vi "集成干预测试数据存储.vi"(8 "error in (no error)":errorcluster, 11 "存储变量":T1) -> (0 "error out":errorcluster)   [LabVIEW 2016, in "PLC.lvlib"]
uses:
  PLC.lvlib
  <vilib>/Utility/sysdir.llb/System Directory Type.ctl
  <vilib>/addons/database/Connection.llb/DB Tools Open Connec (String).vi
  <vilib>/addons/database/NI_Database_API.lvlib
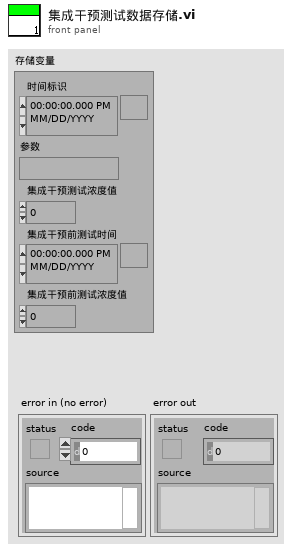
[diagram p1: front panel]
types:
  T1 = cluster{"时间标识":timestamp, "参数":string, "集成干预测试浓度值":dbl, "集成干预前测试时间":timestamp, "集成干预前测试浓度值":dbl}
  T2 = typedef "System Directory Type.ctl" = i32
  T3 = typedef "NI_Database_API.lvlib/Conn ObjectReference.ctl" = refnum<k1>
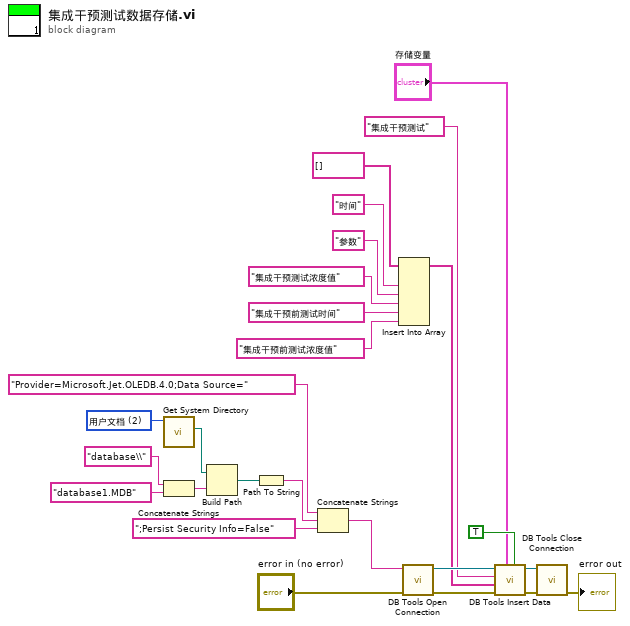
[diagram p0: block diagram]
diagram:
  w23 = T2 2 items=["用户目录"=0, "用户桌面"=1, "用户文档"=2, "用户应用程序数据"=3, "用户设置"=4, "用户临时目录"=5, "公共文档"=6, "公共应用程序数据"=7, "公共设置"=8, "公共缓存"=13, "系统核心库"=9, "系统安装库"=10, "应用程序文件"=11, "启动盘根目录"=12] ("system directory type")
  n1 = call <vilib>:"Get System Directory.vi"("system directory type"=w23) -> ("system directory"=w21:path)  [unwired: 10 in]
  n2 = Concatenate Strings("database\\" ("condition"), "database1.MDB" ("condition")) -> (w15:string)
  n3 = Build Path(base path=w21, name or relative path=w15) -> (appended path=w20:path)
  n4 = Path To String(path=w20) -> (string=w19:string)
  n5 = Concatenate Strings("Provider=Microsoft.Jet.OLEDB.4.0;Data Source=" ("condition"), w19, ";Persist Security Info=False" ("condition")) -> (w17:string)
  n6 = Insert Into Array(array=string[] [] ("columns"), new element #1="时间" ("新元素/子数组"), new element #2="参数" ("新元素/子数组"), new element #3="集成干预测试浓度值" ("新元素/子数组"), new element #4="集成干预前测试时间" ("新元素/子数组"), new element #5="集成干预前测试浓度值" ("新元素/子数组")) -> (w6:string[])  [unwired: 1 in]
  n7 = call-poly <vilib>:"DB Tools Open Connection.vi"("error in (no error)"="error in (no error)", "connection information"=w17) -> ("error out"=w13:errorcluster, "connection reference"=w14:T3)  [unwired: 6 in]
  n8 = call <vilib>:"DB Tools Insert Data.vi"("create table? (F)"=TRUE, "data"="存储变量", "error in (no error)"=w13, "columns"=w6, "table"="集成干预测试", "connection reference"=w14) -> ("error out"=w25:errorcluster, "connection reference out"=w26:T3)  [unwired: 4 in]
  n9 = call <vilib>:"DB Tools Close Connection.vi"("error in (no error)"=w25, "connection reference"=w26) -> ("error out"=→"error out":errorcluster)  [unwired: 5 in]
